vi "SubVI_Flash Detection #.vi"(0 "Image In":T2, 1 "Edge Options":T3={"Edge Polarity"=0, "Kernel Size"=3, "Width"=3, "Minimum Edge Strength"=10.0, "Interpolation Type"=enum."Bilinear Fixed", "Data Processing Method"=enum."Average"} {"Edge Polarity" items=["All Edges", "Rising Edges", "Falling Edges"]; "Minimum Edge Strength" format="%.2f"; "Width" step=2; "Kernel Size" step=2}, 5 "ROI Descriptor":T5 {"Contours"."Type" items=["No Selection", "Point", "Line", "Rectangle", "Oval", "Polygon", "Free", "Annulus", "Unused2", "Unused3", "Broken Line", "Free Hand Line", "Rotated Rectangle"]}, 7 "Flash Detection":enum16{"Datum C", "Arc"}(ring), 9 "Step Size":i32=5, 11 "Error in":errorcluster, 12 "Scan Direction":u16(ring) items=["Left To Right", "Right To Left", "Top To Bottom", "Bottom To Top"]) -> (4 "Image Out":T2, 6 "Distance":dbl, 8 "Perpendicular Line":T1, 10 "Fit Line":T1, 15 "Error out":errorcluster)   [LabVIEW 2013]
uses:
  <vilib>/vision/Measure.llb/Edge Options.ctl
  <vilib>/vision/Measure.llb/Edge Polarity.ctl
  <vilib>/vision/Image Controls.llb/IMAQ Image.ctl
  <vilib>/vision/NI_Vision_Development_Module.lvlib
  <vilib>/Analysis/NI_AALPro.lvlib
  <vilib>/Analysis/6fits.llb/Curve Fitting Criteria.ctl
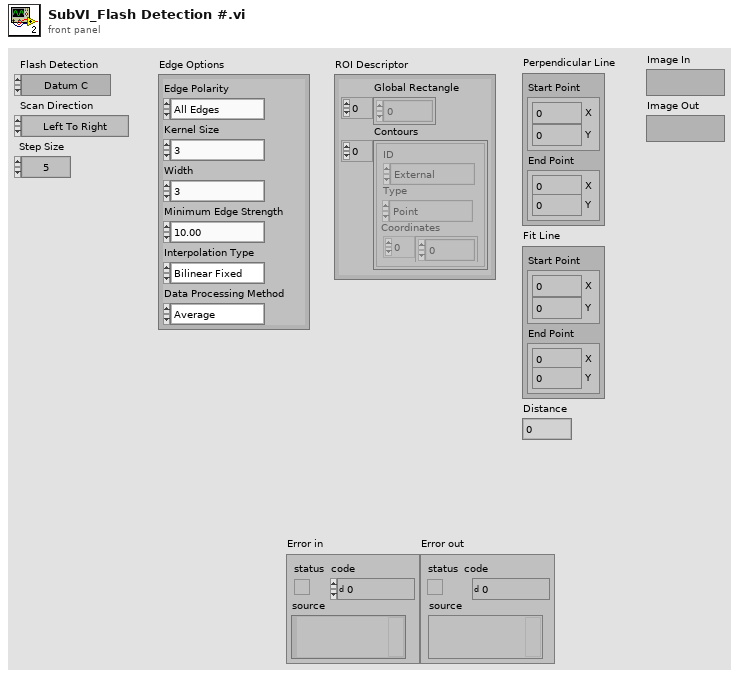
[diagram p1: front panel]
types:
  T1 = cluster{"Start Point":cluster{"X":i32, "Y":i32}, "End Point":cluster{"X":i32, "Y":i32}}
  T2 = typedef "IMAQ Image.ctl" = refnum<image>
  T3 = typedef "Edge Options.ctl" = cluster{"Edge Polarity":T4, "Kernel Size":u32, "Width":u32, "Minimum Edge Strength":sgl, "Interpolation Type":enum32{"Zero Order", "Bilinear", "Quadratic", "Cubic", "Bilinear Fixed"}, "Data Processing Method":enum32{"Average", "Median"}}
  T4 = typedef "Edge Polarity.ctl" = u32
  T5 = cluster{"Global Rectangle":i32[], "Contours":cluster{"ID":enum32{"External", "Internal"}, "Type":u32, "Coordinates":i32[]}[]}
  T6 = enum16{"Get First Edge", "Get First + Last Edge", "Get All Edges", "Get Best Edge"}
  T7 = cluster{"[0]":cluster{"X":i32, "Y":i32}, "Location (Pixel)":cluster{"X":i32, "Y":i32}}
  T8 = typedef "Edge New.ctl" = cluster{"Location (Pixel)":cluster{"X":sgl, "Y":sgl}, "Location (Real-World)":cluster{"X":sgl, "Y":sgl}, "Distance (Pixel)":dbl, "Distance (Real-World)":dbl, "Strength":dbl, "Noise":dbl, "Rising?":bool}
  T9 = typedef "NI_AALPro.lvlib/Curve Fitting Criteria.ctl" = u16
  T10 = cluster{cluster{"X":sgl, "Numeric":sgl}, cluster{"X":sgl, "Numeric":sgl}}
  T11 = cluster{"Point 1":cluster{"X":sgl, "Y":sgl}, "Point 2":cluster{"X":sgl, "Y":sgl}}
  T12 = cluster{"Point 1":cluster{"X":i32, "Y":i32}, "Point 2":cluster{"X":i32, "Y":i32}}
  T13 = cluster{"[0]":cluster{"X":sgl, "Y":sgl}, "[1]":cluster{"X":sgl, "Y":sgl}}
  T14 = cluster{"[0]":cluster{"X":i32, "Y":i32}, "[1]":cluster{"X":i32, "Y":i32}}
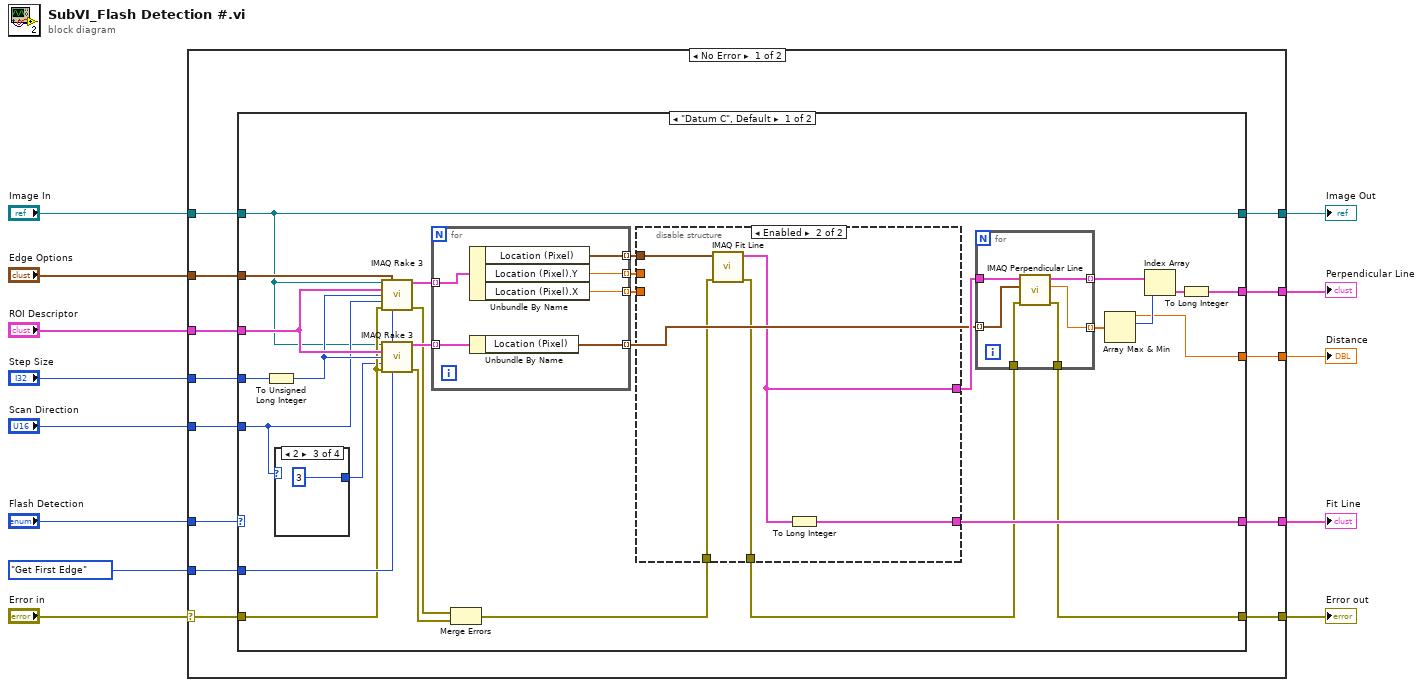
[diagram p0: block diagram]
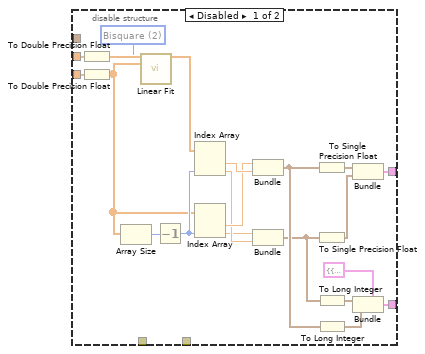
[diagram p2: hidden frame]
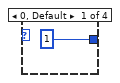
[diagram p3: hidden frame]
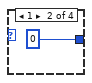
[diagram p4: hidden frame]
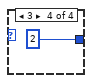
[diagram p5: hidden frame]
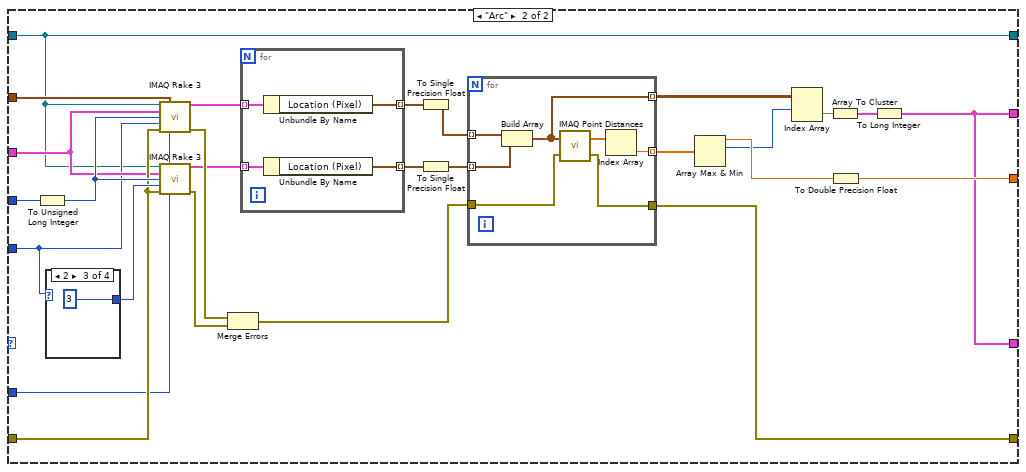
[diagram p6: hidden frame]
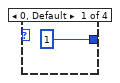
[diagram p7: hidden frame]
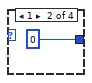
[diagram p8: hidden frame]
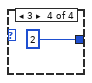
[diagram p9: hidden frame]
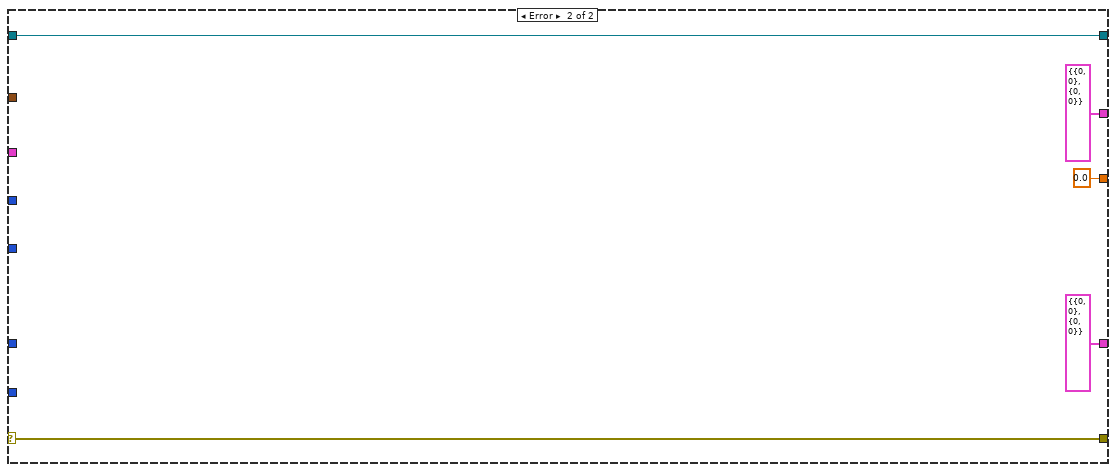
[diagram p10: hidden frame]
diagram:
  n1 = case shown="No Error" "Error in" {
    selector: "Error in" -> [w14 w139]
    tunnel: "Flash Detection" -> [w26 _]
    tunnel: T6."Get First Edge" ("Process") -> [w25 _]
    tunnel: "Scan Direction" -> [w24 _]
    tunnel: "Step Size" -> [w23 _]
    tunnel: "ROI Descriptor" -> [w22 _]
    tunnel: "Edge Options" -> [w21 _]
    tunnel: "Image In" -> [w20 w143]
    tunnel: [w19 w143] -> w6
    tunnel: [w18 T7 {"[0]"={"X"=0, "Y"=0}, "Location (Pixel)"={"X"=0, "Y"=0}}] -> w5
    tunnel: [w17 T1 {"Start Point"={"X"=0, "Y"=0}, "End Point"={"X"=0, "Y"=0}} ("Fit Line")] -> w4
    tunnel: [w16 0.0] -> w3
    tunnel: [w15 w139] -> w2
    frame No Error {
      n2 = case shown="\"Datum C\", Default" w26 {
        tunnel: w20 -> [w29 w98]
        tunnel: w25 -> [w41 w109]
        tunnel: w24 -> [w33 w103]
        tunnel: w23 -> [w40 w108]
        tunnel: w22 -> [w42 w107]
        tunnel: w21 -> [w31 w106]
        tunnel: [w29 w98] -> w19
        tunnel: [w45 w99] -> w18
        tunnel: [w44 w99] -> w17
        tunnel: [w38 w105] -> w16
        tunnel: w14 -> [w37 w110]
        tunnel: [w34 w104] -> w15
        frame "Datum C", Default {
          n3 = To Unsigned Long Integer(number=w40) -> (unsigned 32bit integer=w39:u32)
          n4 = case shown="2" w33 {
            tunnel: [u16 1 u16 0 u16 3 u16 2] -> w32
            frame 0, Default {
            }
            frame 1 {
            }
            frame 2 {
            }
            frame 3 {
            }
          }
          n5 = call "IMAQ Rake 3"("Image"=w29, "Edge Options"=w31, "ROI Descriptor"=w42, "Step Size"=w39, "Scan Direction"=w33, "error in (no error)"=w37, "Process"=w41) -> ("First Edges"=w54:T8[], "error out"=w36:errorcluster)  [unwired: 5 in, 2 out]
          n6 = call "IMAQ Rake 3"("Image"=w29, "Edge Options"=w31, "ROI Descriptor"=w42, "Step Size"=w39, "Scan Direction"=w32, "error in (no error)"=w37, "Process"=w41) -> ("First Edges"=w43:T8[], "error out"=w35:errorcluster)  [unwired: 5 in, 2 out]
          n7 = for {
            tunnel: w54 -> [w92] mode=indexing
            tunnel: [w96] -> w53 mode=indexing
            tunnel: [w95] -> w51 mode=indexing
            tunnel: [w93] -> w49 mode=indexing
            tunnel: w43 -> [w94] mode=indexing
            tunnel: [w91] -> w30 mode=indexing
            n8 = Unbundle By Name(w92) -> ("Location (Pixel)"=w91:cluster{"X":sgl, "Y":sgl}, "Location (Pixel).Y"=w96:sgl, "Location (Pixel).X"=w95:sgl)
            n9 = Unbundle By Name(w94) -> ("Location (Pixel)"=w93:cluster{"X":sgl, "Y":sgl})
          }
          n10 = Merge Errors(w36, w35) -> (w28:errorcluster)
          n11 = disable-structure shown="Enabled" {
            disable-tunnel: w53 -> [w75 _]
            disable-tunnel: w51 -> [w74 _]
            disable-tunnel: [w73 w78] -> w50
            disable-tunnel: [w67 w79] -> w44
            disable-tunnel: w30 -> [_ w80]
            disable-tunnel: w28 -> [_ w77]
            disable-tunnel: [_ w76] -> w27
            frame Disabled {
              w55 = T9 2 items=["Least Square", "Least Absolute Residual", "Bisquare"] ("method")
              n12 = To Double Precision Float(number=w75) -> (double precision float=w66:dbl[])
              n13 = To Double Precision Float(number=w74) -> (double precision float=w63:dbl[])
              n14 = Array Size(array=w63) -> (size(s)=w65:i32)
              n15 = call <vilib>:"Linear Fit.vi"("Y"=w66, "X"=w63, "method"=w55) -> ("Best Linear Fit"=w62:dbl[])  [unwired: 8 in, 4 out]
              n16 = Decrement(x=w65) -> (x-1=w64:i32)
              n17 = Index Array(array=w62, index #2=w64) -> (element #1=w59:dbl, element #2=w57:dbl)  [unwired: 1 in]
              n18 = Index Array(array=w63, index #2=w64) -> (element #1=w58:dbl, element #2=w56:dbl)  [unwired: 1 in]
              n19 = Bundle("X"=w58, "Numeric"=w59) -> (w72:cluster{"X":dbl, "Numeric":dbl})  [unwired: 1 in]
              n20 = Bundle("X"=w56, "Numeric"=w57) -> (w71:cluster{"X":dbl, "Numeric":dbl})  [unwired: 1 in]
              n21 = To Single Precision Float(number=w72) -> (single precision float=w60:cluster{"X":sgl, "Numeric":sgl})
              n22 = To Single Precision Float(number=w71) -> (single precision float=w61:cluster{"X":sgl, "Numeric":sgl})
              n23 = To Long Integer(number=w71) -> (32bit integer=w70:cluster{"X":i32, "Numeric":i32})
              n24 = To Long Integer(number=w72) -> (32bit integer=w69:cluster{"X":i32, "Numeric":i32})
              n25 = Bundle(w60, w61) -> (w73:T10)  [unwired: 1 in]
              n26 = Bundle(cluster=T1 {"Start Point"={"X"=0, "Y"=0}, "End Point"={"X"=0, "Y"=0}} ("Fit Line"), "Start Point"=w70, "End Point"=w69) -> (w67:T1)
            }
            frame Enabled {
              n27 = call "IMAQ Fit Line"("error in (no error)"=w77, "Points"=w80) -> ("error out"=w76:errorcluster, "Line Segment"=w78:T11)  [unwired: 4 in, 4 out]
              n28 = To Long Integer(number=w78) -> (32bit integer=w79:T12)
            }
          }
          n29 = for {
            tunnel: w49 -> [w90] mode=indexing
            tunnel: [w89] -> w48 mode=indexing
            tunnel: [w88] -> w47 mode=indexing
            tunnel: w50 -> [w87]
            tunnel: w27 -> [w86]
            tunnel: [w85] -> w34
            n30 = call "IMAQ Perpendicular Line"("error in (no error)"=w86, "Point"=w90, "Line"=w87) -> ("error out"=w85:errorcluster, "Distance"=w89:dbl, "Perpendicular Line"=w88:T11)  [unwired: 6 in]
          }
          n31 = Array Max & Min(array=w48) -> (max value=w38:dbl, max index (indices)=w52:i32)  [unwired: 2 out]
          n32 = Index Array(array=w47, index=w52) -> (element=w46:T11)
          n33 = To Long Integer(number=w46) -> (32bit integer=w45:T12)
        }
        frame "Arc" {
          n34 = To Unsigned Long Integer(number=w108) -> (unsigned 32bit integer=w113:u32)
          n35 = case shown="2" w103 {
            tunnel: [u16 1 u16 0 u16 3 u16 2] -> w116
            frame 0, Default {
            }
            frame 1 {
            }
            frame 2 {
            }
            frame 3 {
            }
          }
          n36 = call "IMAQ Rake 3"("Image"=w98, "Edge Options"=w106, "ROI Descriptor"=w107, "Step Size"=w113, "Scan Direction"=w103, "error in (no error)"=w110, "Process"=w109) -> ("First Edges"=w111:T8[], "error out"=w114:errorcluster)  [unwired: 5 in, 2 out]
          n37 = call "IMAQ Rake 3"("Image"=w98, "Edge Options"=w106, "ROI Descriptor"=w107, "Step Size"=w113, "Scan Direction"=w116, "error in (no error)"=w110, "Process"=w109) -> ("First Edges"=w112:T8[], "error out"=w115:errorcluster)  [unwired: 5 in, 2 out]
          n38 = Merge Errors(w114, w115) -> (w123:errorcluster)
          n39 = for {
            tunnel: w111 -> [w134] mode=indexing
            tunnel: [w133] -> w97 mode=indexing
            tunnel: [w131] -> w100 mode=indexing
            tunnel: w112 -> [w132] mode=indexing
            n40 = Unbundle By Name(w134) -> ("Location (Pixel)"=w133:cluster{"X":sgl, "Y":sgl})
            n41 = Unbundle By Name(w132) -> ("Location (Pixel)"=w131:cluster{"X":sgl, "Y":sgl})
          }
          n42 = To Single Precision Float(number=w97) -> (single precision float=w101:cluster{"X":sgl, "Y":sgl}[])
          n43 = To Single Precision Float(number=w100) -> (single precision float=w102:cluster{"X":sgl, "Y":sgl}[])
          n44 = for {
            tunnel: w102 -> [w126] mode=indexing
            tunnel: [w130] -> w120 mode=indexing
            tunnel: [w129] -> w119 mode=indexing
            tunnel: w101 -> [w128] mode=indexing
            tunnel: w123 -> [w125]
            tunnel: [w124] -> w104
            n45 = Build Array(w128, w126) -> (w129:cluster{"X":sgl, "Y":sgl}[])
            n46 = call "IMAQ Point Distances"("Points"=w129, "error in (no error)"=w125) -> ("Distances"=w127:sgl[], "error out"=w124:errorcluster)  [unwired: 3 in]
            n47 = Index Array(array=w127) -> (element=w130:sgl)  [unwired: 1 in]
          }
          n48 = Array Max & Min(array=w120) -> (max value=w122:sgl, max index (indices)=w121:i32)  [unwired: 2 out]
          n49 = Index Array(array=w119, index (row)=w121) -> (element=w118:cluster{"X":sgl, "Y":sgl}[])  [unwired: 1 in]
          n50 = Array To Cluster(array=w118) -> (cluster=w117:T13)
          n51 = To Double Precision Float(number=w122) -> (double precision float=w105:dbl)
          n52 = To Long Integer(number=w117) -> (32bit integer=w99:T14)
        }
      }
    }
    frame Error {
    }
  }
  "Image Out" <- w6
  "Perpendicular Line" <- w5
  "Fit Line" <- w4
  "Distance" <- w3
  "Error out" <- w2
